vi "Template.vi"(0 "Notifier Name In":string, 2 "Wait for Finish":bool=TRUE, 11 "Error In":errorcluster) -> (4 "Notifier Name Out":string, 15 "Error Out":errorcluster)   [LabVIEW 2020]
uses:
  Microscopes Type Defs/Microscope Notifier.ctl
  Microscopes Type Defs/Microscope Actions.ctl
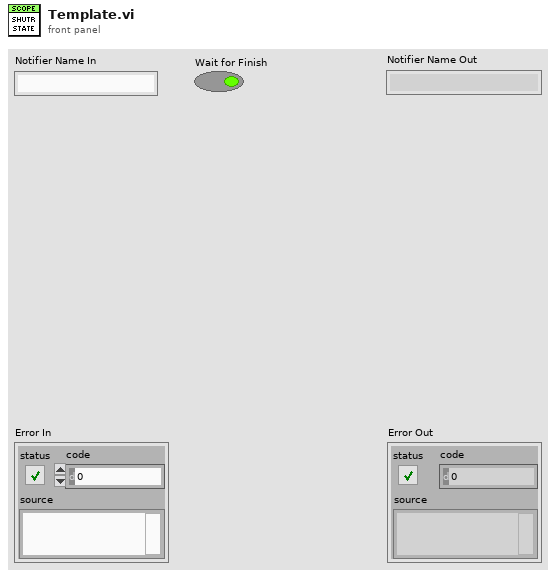
[diagram p1: front panel]
types:
  T1 = typedef "Microscope Notifier.ctl" = cluster{"Actions":T2, "Action Done":bool, "Objective Index":u8, "Objective Z Position (um)":dbl, "Lamp Index":u8, "Lamp State":bool, "Output Port":u8, "Shutter Index":u8, "Shutter State":bool, "Dichroic Wheel Position":u8, "Parameter":string, "Parameter Value":string, "Base Locked?":bool, "Obj Speed":u32, "Obj Acceleration":u32, "Obj Deceleration":u32, "Lamp Power (%)":dbl}
  T2 = typedef "Microscope Actions.ctl" = enum16{"Do Nothing", "Lock Base", "Lock Focus Knob", "Get Objective Index", "Get Objective Z Position", "Get Lamp State", "Get Lamp Power", "Get Output Port", "Get Shutter State", "Get Dichroic Wheel Position", "Set Lamp Index", "Set Shutter Index", "Set Objective Z Position", "Set Lamp State", "Set Lamp Power", "Set Output Port", "Set Shutter State", "Set Dichroic Wheel Position", "Set Objective", "Abort Move", "Set Parameter", "Get Parameter", "Quit"}
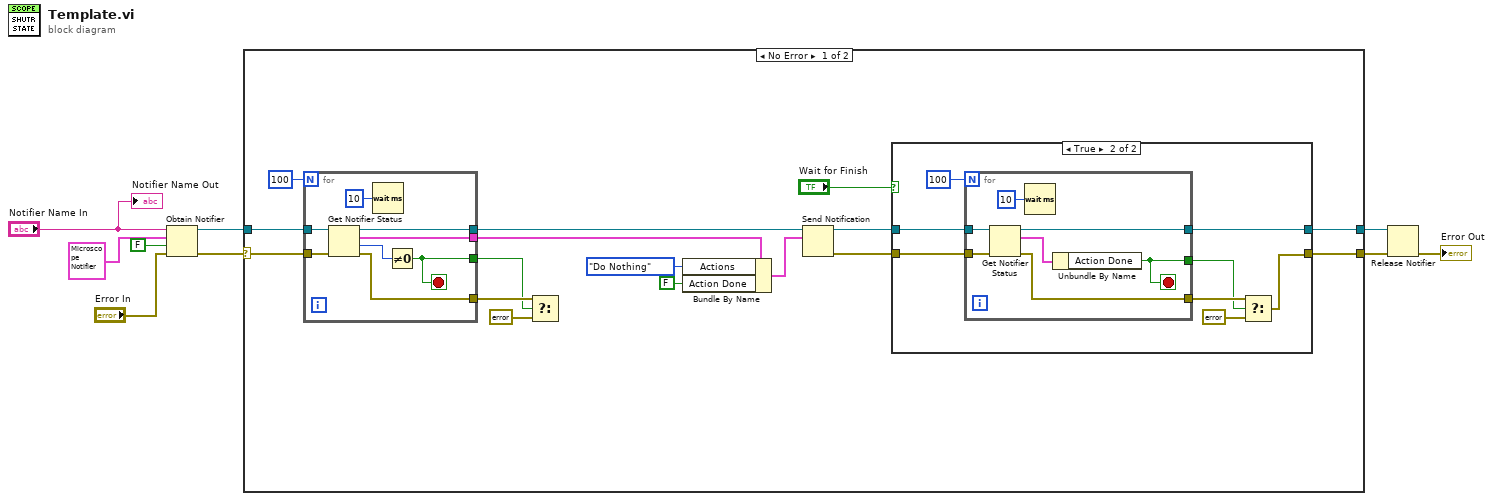
[diagram p0: block diagram]
diagram:
  n1 = Obtain Notifier(name (unnamed)="Notifier Name In", notification data type=T1 {"Actions"=enum."Get Objective Index", "Action Done"=FALSE, "Objective Index"=0, "Objective Z Position (um)"=0.0, "Lamp Index"=0, "Lamp State"=FALSE, "Output Port"=0, "Shutter Index"=0, "Shutter State"=FALSE, "Dichroic Wheel Position"=0, "Parameter"="", "Parameter Value"="", "Base Locked?"=FALSE, "Obj Speed"=0, "Obj Acceleration"=0, "Obj Deceleration"=0, "Lamp Power (%)"=0.0} ("Microscope Notifier"), create if not found? (T)=FALSE, error in (no error)="Error In") -> (notifier out=w6:refnum<notifier>, error out=w7:errorcluster)  [unwired: 1 out]
  n2 = case shown="No Error" w7 {
    selector: w7 -> [w23 w52]
    tunnel: w6 -> [w25 w51]
    tunnel: [w14 w52] -> w2
    tunnel: [w15 w51] -> w3
    frame No Error {
      n3 = for {
        N: 100 -> [_]
        tunnel: w25 -> [w50]
        tunnel: [w48] -> w11
        tunnel: [w46] -> w21
        tunnel: w23 -> [w45]
        tunnel: [w44] -> w12
        tunnel: [w43] -> w22
        stop <- w48 stop-if-true
        n4 = Get Notifier Status(notifier=w50, error in (no error)=w45) -> (notifier out=w46:refnum<notifier>, current notification=w43:T1, # waiting=w49:i32, error out=w44:errorcluster)  [unwired: 1 out]
        n5 = Wait (ms)(milliseconds to wait=u32 10) -> ()  [unwired: 1 out]
        n6 = Not Equal To 0?(x=w49) -> (x != 0?=w48:bool)
      }
      n7 = Select(t=w12, s=w11, f=errorcluster {"status"=TRUE, "code"=0, "source"="IX81 Base Error: Base busy time out."}) -> ()  [unwired: 1 out]
      n8 = Bundle By Name(cluster=w22, "Actions"=Microscope_Actions."Do Nothing", "Action Done"=FALSE) -> (w20:T1)
      n9 = Send Notification(notification=w20, notifier=w21) -> (notifier out=w16:refnum<notifier>, error out=w19:errorcluster)  [unwired: 1 in]
      n10 = case shown="True" "Wait for Finish" {
        tunnel: w19 -> [w26 w35]
        tunnel: w16 -> [w27 w34]
        tunnel: [w27 w33] -> w15
        tunnel: [w26 w32] -> w14
        frame False {
        }
        frame True {
          n11 = for {
            N: 100 -> [_]
            tunnel: w34 -> [w42]
            tunnel: [w40] -> w33
            tunnel: w35 -> [w39]
            tunnel: [w38] -> w30
            tunnel: [w36] -> w29
            stop <- w36 stop-if-true
            n12 = Get Notifier Status(notifier=w42, error in (no error)=w39) -> (notifier out=w40:refnum<notifier>, current notification=w37:T1, error out=w38:errorcluster)  [unwired: 2 out]
            n13 = Wait (ms)(milliseconds to wait=u32 10) -> ()  [unwired: 1 out]
            n14 = Unbundle By Name(w37) -> ("Action Done"=w36:bool)
          }
          n15 = Select(t=w30, s=w29, f=errorcluster {"status"=TRUE, "code"=0, "source"="IX81 Base Error: Action didn't complete."}) -> (s? t:f=w32:errorcluster)
        }
      }
    }
    frame Error {
    }
  }
  n16 = Release Notifier(notifier=w3, error in (no error)=w2) -> (error out=→"Error Out":errorcluster)  [unwired: 1 in, 2 out]
  "Notifier Name Out" <- "Notifier Name In"
